vi "FTW-JSON-Object-SetElement-Bool.vi"(0 "JSON Object":refnum<class "FTW-JSON.lvclass">, 5 "Key":string, 7 "Value":bool, 11 "error in":errorcluster) -> (4 "JSON Object out":refnum<class "FTW-JSON.lvclass">, 15 "error out":errorcluster)   [LabVIEW 2013, in "FTW-JSON.lvclass"]
uses:
  FTW-JSON.lvclass
  FTW-JSON.lvclass/FTW-JSON.ctl
panel:
  # "Inputs"
  # "Outputs"
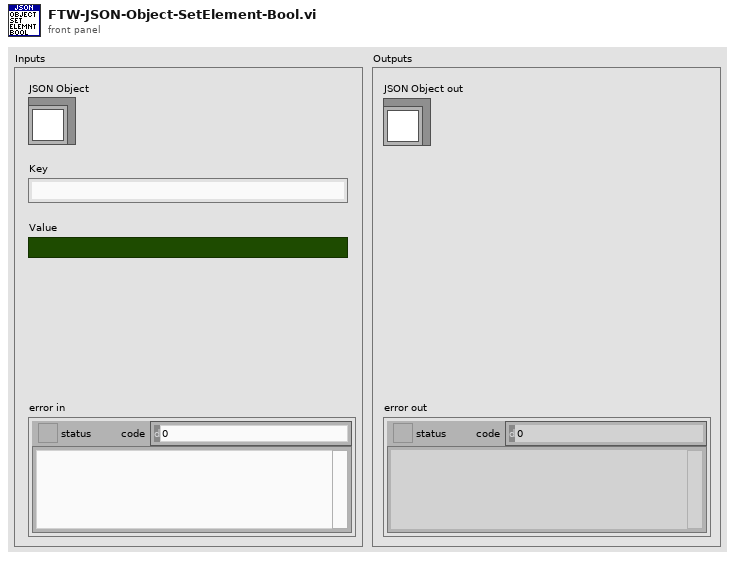
[diagram p1: front panel]
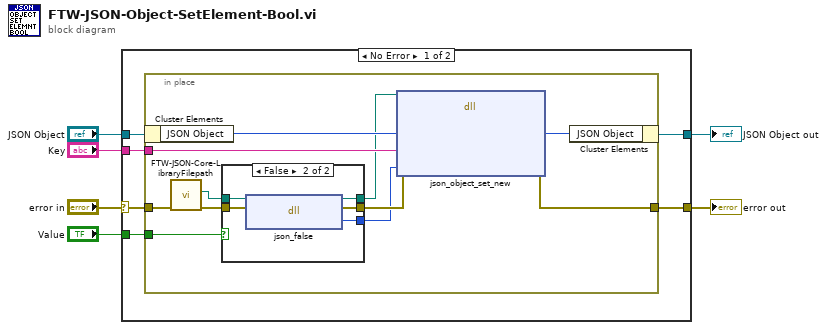
[diagram p0: block diagram]
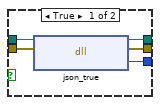
[diagram p2: hidden frame]
diagram:
  n1 = case shown="No Error" "error in" {
    selector: "error in" -> [w10 w35]
    tunnel: [w9 w35] -> w6
    tunnel: [w8 w34] -> w4
    tunnel: "JSON Object" -> [w12 w34]
    tunnel: "Key" -> [w11 _]
    tunnel: "Value" -> [w7 _]
    frame No Error {
      n2 = in-place {
        in-place-border: w10 -> [w23]
        in-place-border: [w22] -> w9
        in-place-border: w11 -> [w19]
        in-place-border: w7 -> [w13]
        n3 = in-place-cluster #1(w12) -> ("JSON Object"=w21:i64)
        n4 = call "FTW-JSON-Core-LibraryFilepath.vi"("error in"=w23) -> ("error out"=w16:errorcluster, "JSON Library Filepath"=w18:path)  [unwired: 9 in]
        n5 = case shown="False" w13 {
          tunnel: w18 -> [w28 w33]
          tunnel: [w27 w32] -> w17
          tunnel: w16 -> [w26 w31]
          tunnel: [w25 w30] -> w15
          tunnel: [w24 w29] -> w14
          frame True {
            n6 = dll-call lib="?" fn="json_true"(path in=w28, error in=w26) -> (path out=w27:path, error out=w25:errorcluster, "New True Value"=w24:i64)  [unwired: 1 in]
          }
          frame False {
            n7 = dll-call lib="?" fn="json_false"(path in=w33, error in=w31) -> (path out=w32:path, error out=w30:errorcluster, "New False Value"=w29:i64)  [unwired: 1 in]
          }
        }
        n8 = dll-call lib="?" fn="json_object_set_new"(path in=w17, error in=w15, "JSON Object Pointer"=w21, "Key"=w19, "New JSON Object"=w14) -> (error out=w22:errorcluster, "JSON Object Pointer"=w20:i64)  [unwired: 4 in, 1 out]
        n9 = in-place-cluster #1("JSON Object"=w20) -> (w8:refnum<class "FTW-JSON.lvclass">)
      }
    }
    frame Error {
    }
  }
  "error out" <- w6
  "JSON Object out" <- w4
